vi "charging.vi"(0 "E in":dbl, 1 "R in":dbl, 2 "C in":dbl) -> (6 "TIME = 9":dbl format="%#_3e", 7 "VC T = 10":dbl format="%#_3e", 8 "TIME = 8":dbl format="%#_3e", 9 "VC T = 9":dbl format="%#_3e", 10 "Time Const 2":dbl, 11 "VC T = 8":dbl format="%#_3e", 12 "TIME = 10":dbl format="%#_3e", 13 "VC T = 7":dbl format="%#_3e", 14 "TIME = 7":dbl format="%#_3e", 15 "TIME = 11":dbl format="%#_3e", 16 "TIME = 6":dbl format="%#_3e", 17 "VC T = 11":dbl format="%#_3e", 18 "VC T = 6":dbl format="%#_3e")   [LabVIEW 2018]
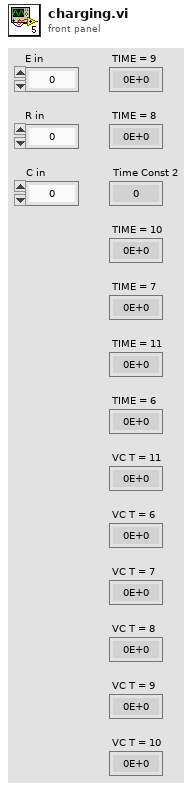
[diagram p1: front panel]
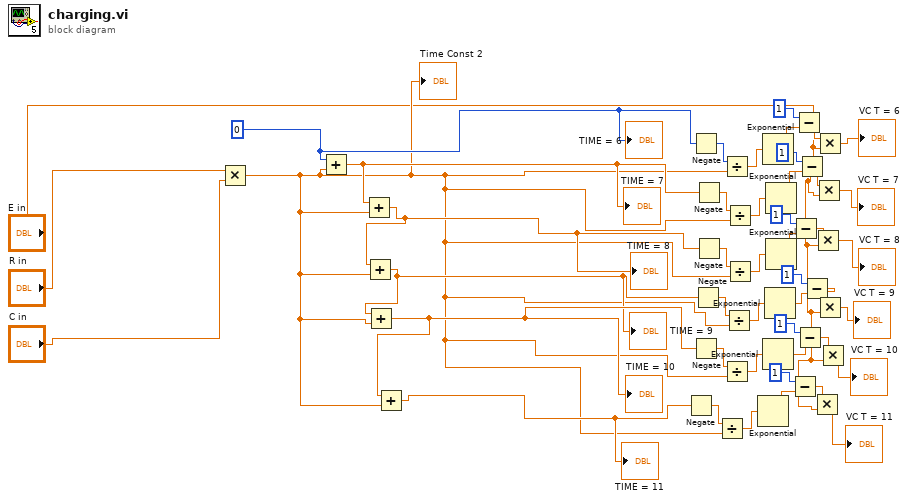
[diagram p0: block diagram]
diagram:
  w23 = 0
  n1 = Multiply(x="R in", y="C in") -> (x*y=w22:dbl)
  "Time Const 2" <- w22
  n2 = Add(x=w23, y=w22) -> (x+y=w24:dbl)
  "TIME = 7" <- w24
  n3 = Add(x=w24, y=w22) -> (x+y=w25:dbl)
  "TIME = 8" <- w25
  n4 = Add(x=w25, y=w22) -> (x+y=w26:dbl)
  "TIME = 9" <- w26
  n5 = Add(x=w26, y=w22) -> (x+y=w27:dbl)
  "TIME = 10" <- w27
  n6 = Add(x=w27, y=w22) -> (x+y=w28:dbl)
  "TIME = 11" <- w28
  n7 = Negate(x=w28) -> (-x=w11:dbl)
  n8 = Negate(x=w23) -> (-x=w1:i32)
  n9 = Negate(x=w27) -> (-x=w9:dbl)
  n10 = Negate(x=w26) -> (-x=w7:dbl)
  n11 = Negate(x=w24) -> (-x=w3:dbl)
  n12 = Negate(x=w25) -> (-x=w5:dbl)
  n13 = Divide(x=w11, y=w22) -> (x/y=w12:dbl)
  n14 = Divide(x=w1, y=w22) -> (x/y=w2:dbl)
  n15 = Divide(x=w9, y=w22) -> (x/y=w10:dbl)
  n16 = Divide(x=w7, y=w22) -> (x/y=w8:dbl)
  n17 = Divide(x=w3, y=w22) -> (x/y=w4:dbl)
  n18 = Divide(x=w5, y=w22) -> (x/y=w6:dbl)
  n19 = Exponential(1:w12) -> (0:w31:dbl)
  n20 = Exponential(1:w2) -> (0:w46:dbl)
  n21 = Exponential(1:w10) -> (0:w35:dbl)
  n22 = Exponential(1:w8) -> (0:w38:dbl)
  n23 = Exponential(1:w4) -> (0:w44:dbl)
  n24 = Exponential(1:w6) -> (0:w41:dbl)
  n25 = Subtract(x=1, y=w31) -> (x-y=w32:dbl)
  n26 = Subtract(x=1, y=w41) -> (x-y=w40:dbl)
  n27 = Subtract(x=1, y=w46) -> (x-y=w45:dbl)
  n28 = Subtract(x=1, y=w35) -> (x-y=w34:dbl)
  n29 = Subtract(x=1, y=w44) -> (x-y=w43:dbl)
  n30 = Subtract(x=1, y=w38) -> (x-y=w37:dbl)
  n31 = Multiply(x=w32, y="E in") -> (x*y=→"VC T = 11":dbl)
  n32 = Multiply(x=w40, y="E in") -> (x*y=→"VC T = 8":dbl)
  n33 = Multiply(x=w43, y="E in") -> (x*y=→"VC T = 7":dbl)
  n34 = Multiply(x=w45, y="E in") -> (x*y=→"VC T = 6":dbl)
  n35 = Multiply(x=w37, y="E in") -> (x*y=→"VC T = 9":dbl)
  n36 = Multiply(x=w34, y="E in") -> (x*y=→"VC T = 10":dbl)
  "TIME = 6" <- w23
